vi "Create Phrase ASCII with Unit or Greek Letter.vi"(0 "Text":string, 2 "PDF Report IN":refnum<class "PDF Report Class.lvclass">, 7 "Cell Font Ref":refnum<k24>, 11 "error in (no error)":errorcluster) -> (8 "Phrase refnum":refnum<k24>, 15 "error out":errorcluster)   [LabVIEW 2020, in "Exaprom PDF.lvlib"]
doc: "Developed by Jean-Marc Simard\nCopyright © 2012, Exaprom Inc.\nAll rights reserved.\nLicense: BSD\n\nWith iTextSharp 4.1.6 (http://itextsharp.sourceforge.net)\nunder Mozilla Public License Version 1.1\n(http://www.mozilla.org/MPL/MPL-1.1.html)"
uses:
  <userlib>/labview-PDF-writer-master/Exaprom PDF.lvlib
  C:/Program Files (x86)/National Instruments/LabVIEW 2020/user.lib/labview-PDF-writer-master/DLL/itextsharp.dll
  DLL/itextsharp.dll
  <userlib>/labview-PDF-writer-master/LV Class/PDF Report Class/PDF Report Class.lvclass
  <userlib>/labview-PDF-writer-master/LV Class/Fonts Class/Font Class.lvclass
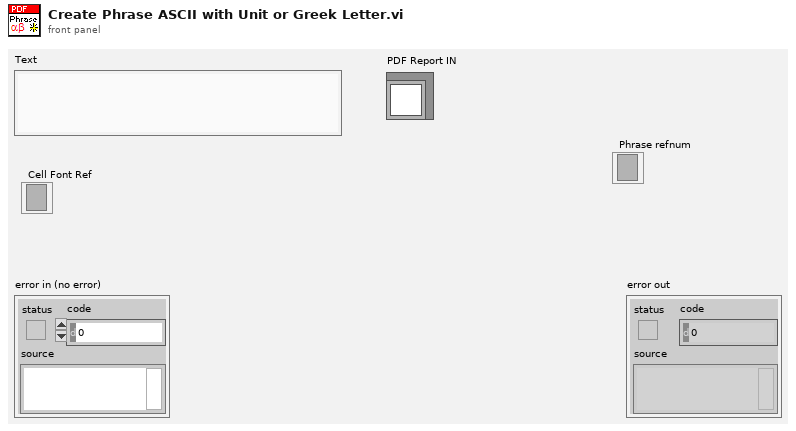
[diagram p1: front panel]
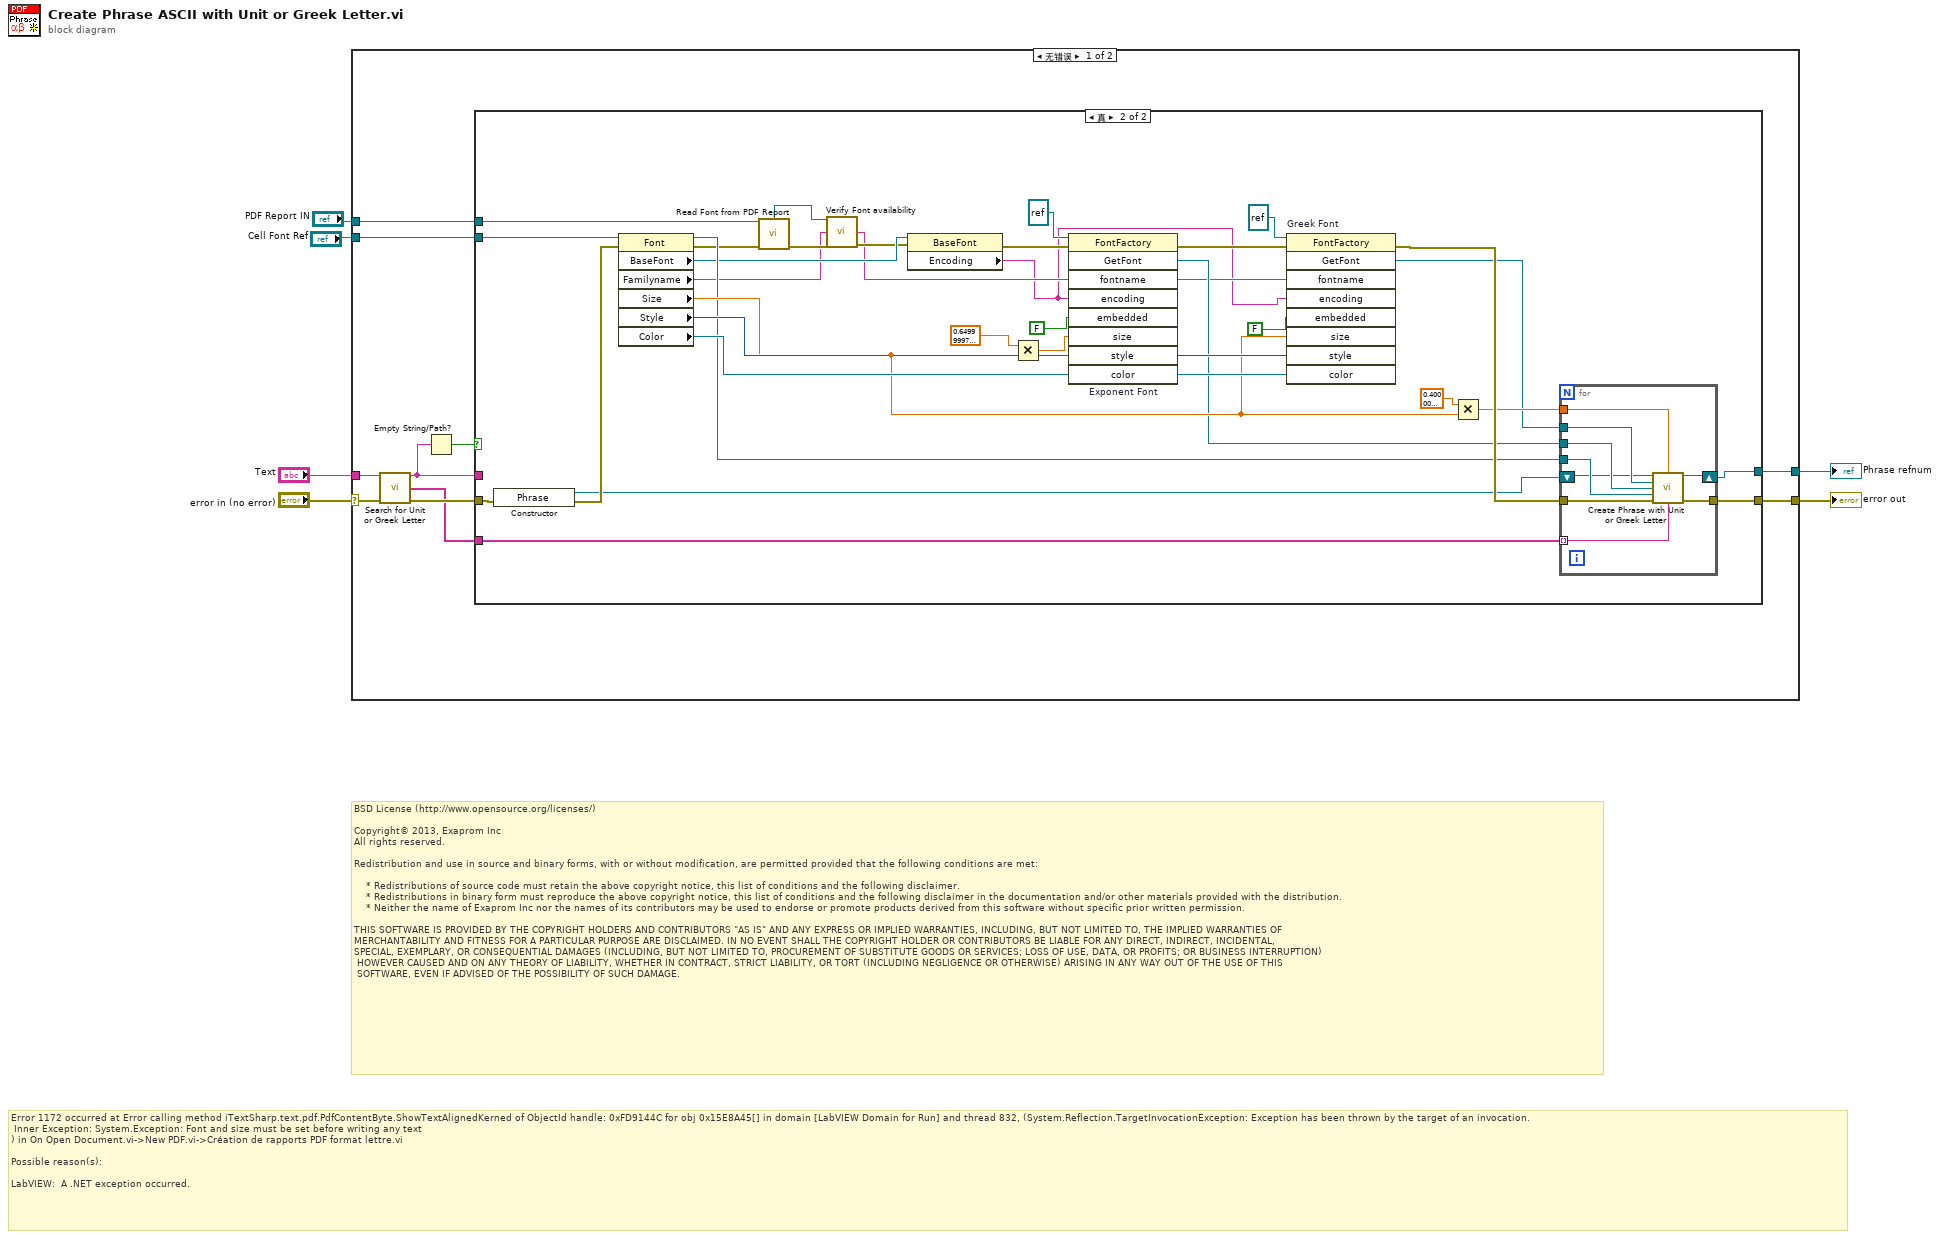
[diagram p0: block diagram]
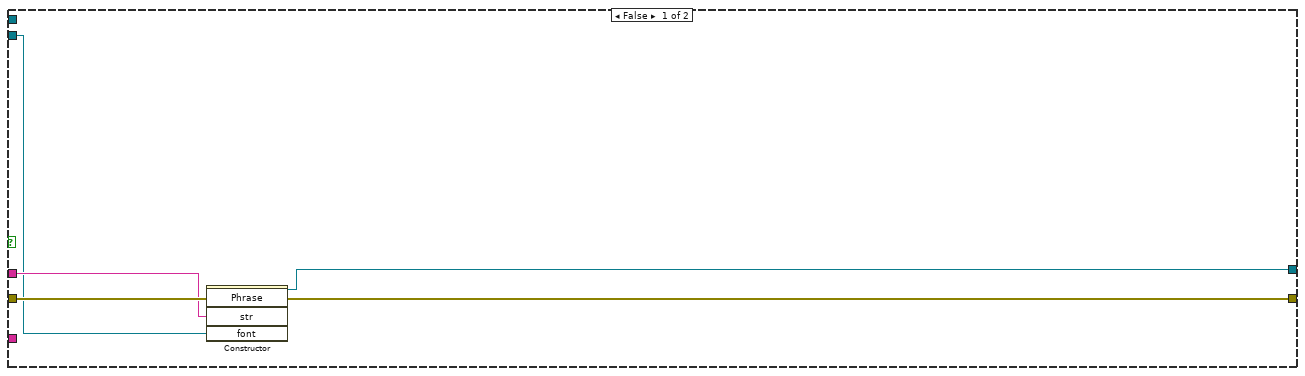
[diagram p2: hidden frame]
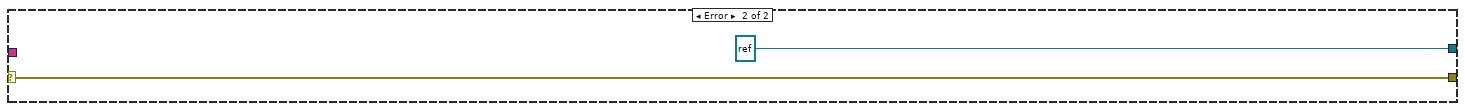
[diagram p3: hidden frame]
diagram:
  # "Error 1172 occurred at Error calling method iTextSharp.text.pdf.PdfContentByte.ShowTextAlignedKerned of ObjectId handle: 0xFD9144C for obj 0x15E8A45[] in domain [LabVIEW Domain for Run] and thread 832, (System.Reflection.TargetInvocationException: Exception has been thrown by the target of an invocation.\n\tInner Exception: System.Exception: Font and size must be set before writing any text\n) in On Open Document.vi->New PDF.vi->Création de rapports PDF format lettre.vi\n\nPossible reason(s):\n\nLabVIEW:  A .NET exception occurred."
  # "BSD License (http://www.opensource.org/licenses/)\n\nCopyright© 2013, Exaprom Inc\nAll rights reserved.\n\nRedistribution and use in source and binary forms, with or without modification, are permitted provided that the following conditions are met:\n\n    * Redistributions of source code must retain the above copyright notice, this list of conditions and the following disclaimer.\n    * Redistributions in binary form must reproduce the above copyright notice, this list of conditions and the following disclaimer in the documentation and/or other materials provided with the distribution.\n    * Neither the name of Exaprom Inc nor the names of its contributors may be used to endorse or promote products derived from this software without specific prior written permission.\n\nTHIS SOFTWARE IS PROVIDED BY THE COPYRIGHT HOLDERS AND CONTRIBUTORS \"AS IS\" AND ANY EXPRESS OR IMPLIED WARRANTIES, INCLUDING, BUT NOT LIMITED TO, THE IMPLIED WARRANTIES OF \nMERCHANTABILITY AND FITNESS FOR A PARTICULAR PURPOSE ARE DISCLAIMED. IN NO EVENT SHALL THE COPYRIGHT HOLDER OR CONTRIBUTORS BE LIABLE FOR ANY DIRECT, INDIRECT, INCIDENTAL,\nSPECIAL, EXEMPLARY, OR CONSEQUENTIAL DAMAGES (INCLUDING, BUT NOT LIMITED TO, PROCUREMENT OF SUBSTITUTE GOODS OR SERVICES; LOSS OF USE, DATA, OR PROFITS; OR BUSINESS INTERRUPTION)\n HOWEVER CAUSED AND ON ANY THEORY OF LIABILITY, WHETHER IN CONTRACT, STRICT LIABILITY, OR TORT (INCLUDING NEGLIGENCE OR OTHERWISE) ARISING IN ANY WAY OUT OF THE USE OF THIS\n SOFTWARE, EVEN IF ADVISED OF THE POSSIBILITY OF SUCH DAMAGE."
  n1 = case shown="无错误" "error in (no error)" {
    selector: "error in (no error)" -> [w8 w65]
    tunnel: [w10 refnum<k24> refnum ("new reference")] -> w5
    tunnel: "Text" -> [w16 _]
    tunnel: "Cell Font Ref" -> [w15 _]
    tunnel: [w9 w65] -> w2
    tunnel: "PDF Report IN" -> [w7 _]
    frame No Error {
      n2 = call <userlib>:"Search for Unit or Greek Letter.vi"("Text"=w16, "error in (no error)"=w8) -> ("Text OUT"=w12:string, "Text [ ]"=w11:string[], "error out"=w14:errorcluster)  [unwired: 11 in]
      n3 = Empty String/Path?(string/path=w12) -> (empty?=w13:bool)
      n4 = case shown="真" w13 {
        tunnel: w15 -> [w17 w53]
        tunnel: w14 -> [w21 w33]
        tunnel: w12 -> [w20 _]
        tunnel: w11 -> [_ w41]
        tunnel: [w19 w39] -> w9
        tunnel: [w18 w34] -> w10
        tunnel: w7 -> [_ w28]
        frame False {
          n5 = constructor class="Phrase"(error in=w21, "str"=w20, "font"=w17) -> (reference out=w18:refnum<k24>, error out=w19:errorcluster)  [unwired: 2 in, 3 out]
        }
        frame True {
          n6 = constructor class="Phrase"(error in=w33) -> (reference out=w31:refnum<k24>, error out=w32:errorcluster)  [unwired: 2 in, 1 out]
          n7 = property class="Font"(reference=w53, error in=w32) -> (reference out=w35:refnum<k24>, error out=w29:errorcluster, "BaseFont"=w30:refnum<k24>, "Familyname"=w24:string, "Size"=w43:sgl, "Style"=w44:i32, "Color"=w45:refnum<k24>)
          n8 = call <userlib>:"Read Font from PDF Report.vi"("PDF Report"=w28, "error in (no error)"=w29) -> ("Font Class.lvclass"=w25:refnum<class "Font Class.lvclass">, "error out"=w27:errorcluster)  [unwired: 7 in, 5 out]
          n9 = call <userlib>:"Verify Font availability.vi"("Font IN"=w25, "Font name"=w24, "error in (no error)"=w27) -> ("Font"=w23:string, "error out"=w26:errorcluster)  [unwired: 10 in, 1 out]
          n10 = property class="BaseFont"(reference=w30, error in=w26) -> (error out=w52:errorcluster, "Encoding"=w22:string)  [unwired: 1 out]
          n11 = Multiply(x=sgl 0.65, y=w43) -> (x*y=w51:sgl)
          n12 = invoke on="Exponent Font" class="FontFactory" method="GetFont"(reference=refnum<k24> refnum, error in=w52, "fontname"=w23, "encoding"=w22, "embedded"=FALSE, "size"=w51, "style"=w44, "color"=w45) -> (error out=w47:errorcluster, "GetFont"=w36:refnum<k24>)  [unwired: 1 in, 7 out]
          n13 = invoke on="Greek Font" class="FontFactory" method="GetFont"(reference=refnum<k24> refnum, error in=w47, "fontname"=w23, "encoding"=w22, "embedded"=FALSE, "size"=w43, "style"=w44, "color"=w45) -> (error out=w40:errorcluster, "GetFont"=w37:refnum<k24>)  [unwired: 1 in, 7 out]
          n14 = Multiply(x=sgl 0.4, y=w43) -> (x*y=w38:sgl)
          n15 = for {
            tunnel: w41 -> [w61] mode=indexing
            tunnel: w40 -> [w63]
            tunnel: [w62] -> w39
            tunnel: w38 -> [w60]
            tunnel: w37 -> [w59]
            tunnel: w36 -> [w58]
            tunnel: w35 -> [w57]
            shift-right: [w55] -> w34
            shift-left: w31 -> [w56]
            n16 = call <userlib>:"Create Phrase with Unit or Greek Letter.vi"("Phrase IN"=w56, "Exponent rise"=w60, "Greek Font Ref"=w59, "Exponent Font Ref"=w58, "Cell Font Ref"=w57, "error in (no error)"=w63, "String"=w61) -> ("Phrase OUT reference 2"=w55:refnum<k24>, "error out"=w62:errorcluster)  [unwired: 7 in]
          }
        }
      }
    }
    frame Error {
    }
  }
  "error out" <- w2
  "Phrase refnum" <- w5
